vi "Doc_Builder_Write_BlockDiagram.vi"(10 "input item file path":path, 11 "NI_report in":refnum<class "NI_report.lvclass">) -> (3 "NI_report out":refnum<class "NI_report.lvclass">)   [LabVIEW 2019]
uses:
  <vilib>/Utility/NIReport.llb/NI_report.lvclass
  <vilib>/Utility/NIReport.llb/HTML Report Image Alignment.ctl
  <vilib>/Utility/NIReport.llb/NI_ReportGenerationCore.lvlib
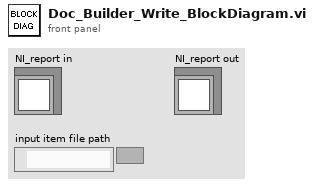
[diagram p1: front panel]
types:
  T1 = typedef "NI_ReportGenerationCore.lvlib/HTML Report Image Alignment.ctl" = enum16{"(default)", "LEFT", "RIGHT", "TOP", "TEXTTOP", "MIDDLE", "ABSMIDDLE", "BASELINE", "BOTTOM", "ABSBOTTOM"}
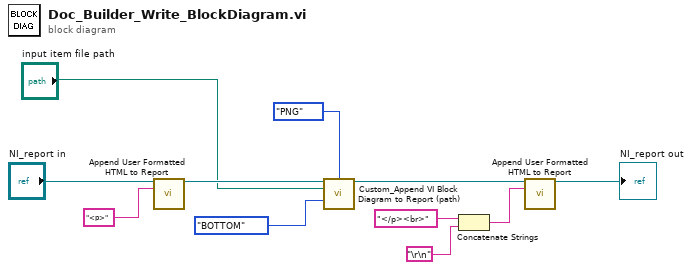
[diagram p0: block diagram]
diagram:
  n1 = call-dynamic "Append User Formatted HTML to Report.vi"("report in"="NI_report in", "HTML text"="<p>" ("text")) -> ("report out"=w4:refnum<class "NI_report.lvclass">)  [unwired: 12 in, 1 out]
  n2 = call "Custom_Append VI Block Diagram to Report (path).vi"("report in"=w4, "image format (jpeg)"=enum32{"PNG", "JPEG", "GIF"}."PNG", "VI"="input item file path", "alignment (default)"=HTML_Report_Image_Alignment."BOTTOM") -> ("report out"=w3:refnum<class "NI_report.lvclass">)  [unwired: 7 in, 4 out]
  n3 = Concatenate Strings("</p><br>" ("text"), "\r\n") -> (w9:string)
  n4 = call-dynamic "Append User Formatted HTML to Report.vi"("report in"=w3, "HTML text"=w9) -> ("report out"=→"NI_report out":refnum<class "NI_report.lvclass">)  [unwired: 12 in, 1 out]
